vi "snake FGV.vi"(0 "X Step Size":fxp<+/-,32,16>, 1 "X End":fxp<+/-,32,16>, 2 "Det Frequency":fxp<+,32,0>=0.9999999997671694, 3 "Traj Frequency":fxp<+,32,0>=0.9999999997671694, 5 "X Start":fxp<+/-,32,16>, 7 "Action":T2, 9 "Y Start":fxp<+/-,32,16>, 11 "Y Step Size":fxp<+/-,32,16>, 12 "Y End":fxp<+/-,32,16>, 13 "Inner Scan axis":T1) -> (4 "X position":fxp<+/-,32,16>, 6 "Y position":fxp<+/-,32,16>, 10 "Number of positions":u32, 15 "Trajectory Complete":bool)   [LabVIEW 2015]
uses:
  Trajectory FGV states.ctl
  Inner Scan axis.ctl
  <vilib>/rvi/Emulation/niFpgaGetClockAttributes.vi
  <vilib>/rvi/Emulation/niFpgaSctlEmulationGetInTimedLoop.vi
  <vilib>/rvi/Emulation/niFpgaEmulationReportErrorSimple.vi
  <vilib>/rvi/Emulation/niFpgaCriticalErrorInLSC.vi
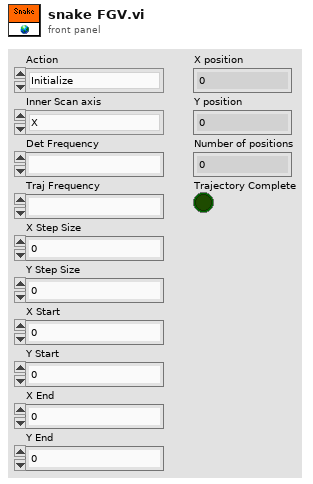
[diagram p1: front panel]
types:
  T1 = typedef "Inner Scan axis.ctl" = enum16{"X", "Y"}
  T2 = typedef "Trajectory FGV states.ctl" = enum16{"Initialize", "Increment"}
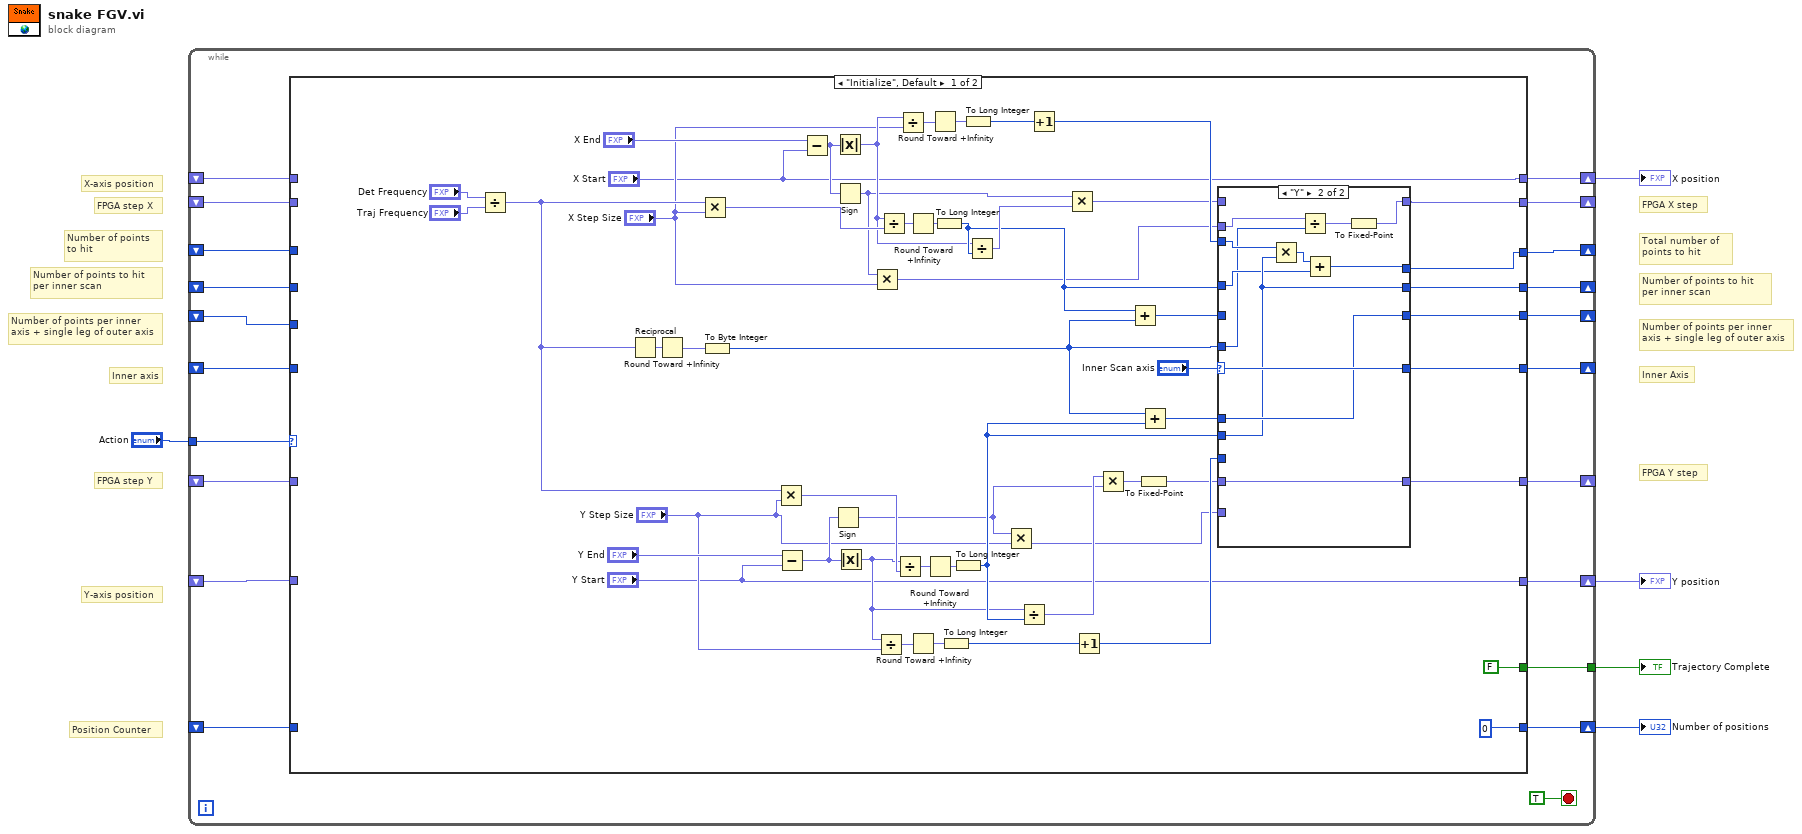
[diagram p0: block diagram]
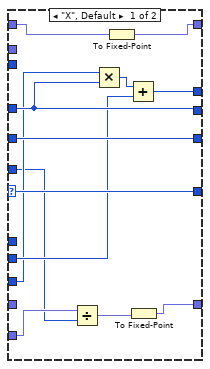
[diagram p2: hidden frame]
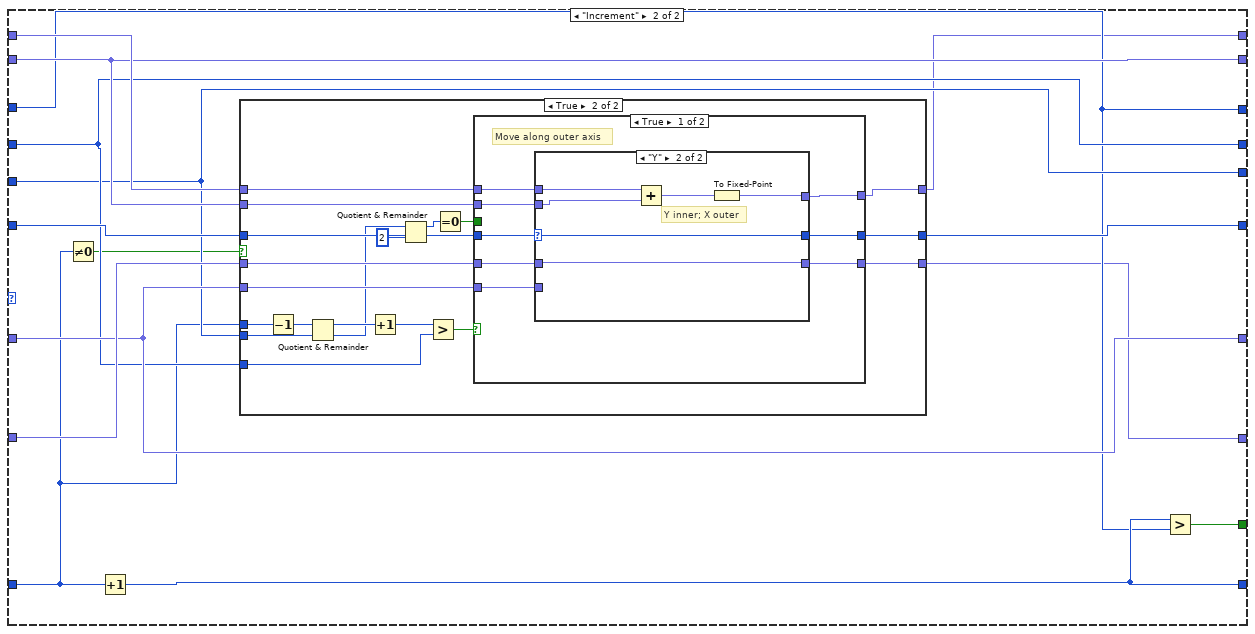
[diagram p3: hidden frame]
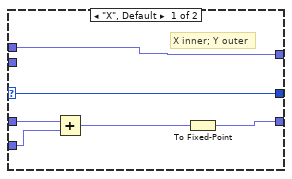
[diagram p5: hidden frame]
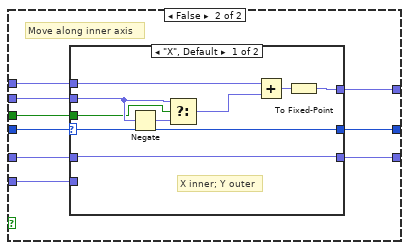
[diagram p6: hidden frame]
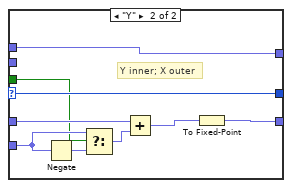
[diagram p7: hidden frame]
diagram:
  # "Number of points per inner \naxis + single leg of outer axis"
  # "Number of points to hit \nper inner scan"
  # "Number of points per inner \naxis + single leg of outer axis"
  # "Inner Axis"
  # "Number of points to hit \nper inner scan"
  # "Inner axis"
  # "FPGA Y step"
  # "FPGA step Y"
  # "Total number of \npoints to hit"
  # "FPGA X step"
  # "Position Counter"
  # "X-axis position"
  # "Y-axis position"
  # "FPGA step X"
  # "Number of points\nto hit"
  n1 = while {
    tunnel: "Action" -> [w25]
    shift-right: [w18] -> _
    shift-left: _ -> [w23]
    shift-right: [w22] -> _
    shift-left: _ -> [w15]
    shift-right: [w6] -> w2
    shift-left: _ -> [w24]
    tunnel: [w21] -> w4
    shift-right: [w20] -> w3
    shift-left: _ -> [w19]
    shift-right: [w17] -> _
    shift-left: _ -> [w16]
    shift-right: [w14] -> _
    shift-left: _ -> [w13]
    shift-right: [w11] -> _
    shift-left: _ -> [w12]
    shift-right: [w10] -> _
    shift-left: _ -> [w9]
    shift-right: [w8] -> w1
    shift-left: _ -> [w7]
    stop <- TRUE stop-if-true
    n2 = case shown="\"Initialize\", Default" w25 {
      tunnel: w7 -> [_ w116]
      tunnel: w24 -> [_ w115]
      tunnel: w23 -> [_ w113]
      tunnel: [w39 w112] -> w17
      tunnel: [w51 w106] -> w22
      tunnel: [FALSE w118] -> w21
      tunnel: [u32 0 w107] -> w20
      tunnel: w19 -> [_ w108]
      tunnel: [w37 w113] -> w18
      tunnel: w16 -> [_ w112]
      tunnel: w15 -> [_ w106]
      tunnel: [w66 w114] -> w14
      tunnel: w13 -> [_ w117]
      tunnel: w12 -> [_ w110]
      tunnel: [w63 w110] -> w11
      tunnel: [w62 w111] -> w10
      tunnel: w9 -> [_ w111]
      tunnel: ["X Start" w105] -> w8
      tunnel: ["Y Start" w104] -> w6
      frame "Initialize", Default {
        n3 = Divide(x="Det Frequency", y="Traj Frequency") -> (x/y=w61:fxp<+,24,8>)
        n4 = Reciprocal(x=w61) -> (1/x=w69:fxp<+,25,17>)
        n5 = Round Toward +Infinity(x=w69) -> (ceil(x): smallest int >= x=w68:fxp<+,17,17>)
        n6 = Multiply(x=w61, y="X Step Size") -> (x*y=w57:fxp<+/-,56,24>)
        n7 = To Byte Integer(number=w68) -> (8bit integer=w34:i8)
        n8 = Multiply(x=w61, y="Y Step Size") -> (x*y=w59:fxp<+/-,56,24>)
        n9 = Subtract(x="Y End", y="Y Start") -> (x-y=w54:fxp<+/-,33,17>)
        n10 = Subtract(x="X End", y="X Start") -> (x-y=w56:fxp<+/-,33,17>)
        n11 = Sign(1:w54) -> (0:w29:fxp<+/-,2,2>)
        n12 = Absolute Value(x=w56) -> (abs(x)=w44:fxp<+,32,16>)
        n13 = Sign(1:w56) -> (0:w27:fxp<+/-,2,2>)
        n14 = Absolute Value(x=w54) -> (abs(x)=w50:fxp<+,32,16>)
        n15 = Multiply(x=w27, y="X Step Size") -> (x*y=w28:fxp<+/-,33,17>)
        n16 = Divide(x=w50, y="Y Step Size") -> (x/y=w49:fxp<+/-,64,33>)
        n17 = Divide(x=w44, y=w57) -> (x/y=w73:fxp<+/-,64,49>)
        n18 = Divide(x=w50, y=w59) -> (x/y=w74:fxp<+/-,64,49>)
        n19 = Divide(x=w44, y="X Step Size") -> (x/y=w46:fxp<+/-,64,33>)
        n20 = Round Toward +Infinity(x=w73) -> (ceil(x): smallest int >= x=w72:fxp<+/-,50,50>)
        n21 = Round Toward +Infinity(x=w49) -> (ceil(x): smallest int >= x=w48:fxp<+/-,34,34>)
        n22 = Round Toward +Infinity(x=w74) -> (ceil(x): smallest int >= x=w60:fxp<+/-,50,50>)
        n23 = Round Toward +Infinity(x=w46) -> (ceil(x): smallest int >= x=w45:fxp<+/-,34,34>)
        n24 = To Long Integer(number=w72) -> (32bit integer=w53:i32)
        n25 = To Long Integer(number=w48) -> (32bit integer=w47:i32)
        n26 = To Long Integer(number=w60) -> (32bit integer=w52:i32)
        n27 = To Long Integer(number=w45) -> (32bit integer=w43:i32)
        n28 = Divide(x=w44, y=w53) -> (x/y=w55:fxp<+/-,64,17>)
        n29 = Multiply(x=w29, y="Y Step Size") -> (x*y=w30:fxp<+/-,33,17>)
        n30 = Divide(x=w50, y=w52) -> (x/y=w58:fxp<+/-,64,17>)
        n31 = Increment(x=w43) -> (x+1=w42:i32)
        n32 = Multiply(x=w27, y=w55) -> (x*y=w38:fxp<+/-,64,18>)
        n33 = Increment(x=w47) -> (x+1=w41:i32)
        n34 = Multiply(x=w58, y=w29) -> (x*y=w40:fxp<+/-,64,18>)
        n35 = Add(x=w53, y=w34) -> (x+y=w65:i32)
        n36 = To Fixed-Point(number=w40) -> (fixed-point=w32:fxp<+/-,24,16>)  [unwired: 1 in]
        n37 = Add(x=w34, y=w52) -> (x+y=w64:i32)
        n38 = case shown="\"Y\"" "Inner Scan axis" {
          selector: "Inner Scan axis" -> [w90 w103]
          tunnel: [w90 w103] -> w66
          tunnel: w65 -> [w91 _]
          tunnel: w64 -> [_ w102]
          tunnel: [w91 w102] -> w63
          tunnel: w52 -> [w86 w100]
          tunnel: w53 -> [w88 w99]
          tunnel: [w88 w100] -> w62
          tunnel: [w87 w97] -> w51
          tunnel: w41 -> [w85 _]
          tunnel: w42 -> [_ w98]
          tunnel: w32 -> [_ w96]
          tunnel: [w81 w96] -> w39
          tunnel: w38 -> [w80 _]
          tunnel: [w79 w92] -> w37
          tunnel: w30 -> [w84 _]
          tunnel: w28 -> [_ w95]
          tunnel: w34 -> [w83 w94]
          frame "X", Default {
            n39 = Divide(x=w84, y=w83) -> (x/y=w82:fxp<+/-,41,17>)
            n40 = Multiply(x=w85, y=w88) -> (x*y=w89:i32)
            n41 = To Fixed-Point(number=w80) -> (fixed-point=w79:fxp<+/-,24,16>)  [unwired: 1 in]
            n42 = Add(x=w89, y=w86) -> (x+y=w87:i32)
            n43 = To Fixed-Point(number=w82) -> (fixed-point=w81:fxp<+/-,24,16>)  [unwired: 1 in]
          }
          frame "Y" {
            n44 = Multiply(x=w98, y=w100) -> (x*y=w101:i32)
            n45 = Divide(x=w95, y=w94) -> (x/y=w93:fxp<+/-,41,17>)
            n46 = Add(x=w101, y=w99) -> (x+y=w97:i32)
            n47 = To Fixed-Point(number=w93) -> (fixed-point=w92:fxp<+/-,24,16>)  [unwired: 1 in]
          }
        }
      }
      frame "Increment" {
        n48 = Not Equal To 0?(x=w108) -> (x != 0?=w109:bool)
        n49 = Increment(x=w108) -> (x+1=w107:u32)
        n50 = case shown="True" w109 {
          tunnel: w117 -> [w121 w140]
          tunnel: w116 -> [w119 w139]
          tunnel: w115 -> [w120 w138]
          tunnel: [w120 w137] -> w104
          tunnel: [w121 w136] -> w114
          tunnel: w108 -> [_ w135]
          tunnel: w113 -> [_ w132]
          tunnel: w112 -> [_ w131]
          tunnel: w111 -> [_ w126]
          tunnel: w110 -> [_ w127]
          tunnel: [w119 w122] -> w105
          frame False {
          }
          frame True {
            n51 = Decrement(x=w135) -> (x-1=w124:u32)
            n52 = Quotient & Remainder(x=w124, y=w127) -> (x-y*floor(x/y)=w134:u32, floor(x/y)=w125:u32)
            n53 = Increment(x=w134) -> (x+1=w123:u32)
            n54 = Quotient & Remainder(x=w125, y=u32 2) -> (x-y*floor(x/y)=w129:u32)  [unwired: 1 out]
            n55 = Greater?(x=w123, y=w126) -> (0:w133:bool)
            n56 = Equal To 0?(x=w129) -> (x = 0?=w128:bool)
            n57 = case shown="True" w133 {
              tunnel: w140 -> [w148 w169]
              tunnel: w139 -> [w147 w168]
              tunnel: [w141 w167] -> w122
              tunnel: w138 -> [w146 w166]
              tunnel: [w145 w165] -> w137
              tunnel: w131 -> [w144 w164]
              tunnel: w132 -> [w143 w163]
              tunnel: [w142 w162] -> w136
              tunnel: w128 -> [_ w161]
              frame True {
                # "Move along outer axis"
                n58 = case shown="\"Y\"" w148 {
                  selector: w148 -> [w153 w157]
                  tunnel: w147 -> [w151 w160]
                  tunnel: w143 -> [_ w159]
                  tunnel: w146 -> [w154 w158]
                  tunnel: [w149 w158] -> w145
                  tunnel: w144 -> [w152 _]
                  tunnel: [w153 w157] -> w142
                  tunnel: [w151 w155] -> w141
                  frame "X", Default {
                    # "X inner; Y outer"
                    n59 = Add(x=w154, y=w152) -> (x+y=w150:fxp<+/-,33,17>)
                    n60 = To Fixed-Point(number=w150) -> (fixed-point=w149:fxp<+/-,24,16>)  [unwired: 1 in]
                  }
                  frame "Y" {
                    # "Y inner; X outer"
                    n61 = Add(x=w160, y=w159) -> (x+y=w156:fxp<+/-,33,17>)
                    n62 = To Fixed-Point(number=w156) -> (fixed-point=w155:fxp<+/-,24,16>)  [unwired: 1 in]
                  }
                }
              }
              frame False {
                # "Move along inner axis"
                n63 = case shown="\"X\", Default" w169 {
                  selector: w169 -> [w176 w186]
                  tunnel: w168 -> [w178 w181]
                  tunnel: w163 -> [w174 _]
                  tunnel: [w170 w181] -> w167
                  tunnel: w166 -> [w177 w187]
                  tunnel: [w177 w179] -> w165
                  tunnel: w164 -> [_ w185]
                  tunnel: [w176 w186] -> w162
                  tunnel: w161 -> [w172 w184]
                  frame "X", Default {
                    # "X inner; Y outer"
                    n64 = Negate(x=w174) -> (-x=w173:fxp<+/-,25,17>)
                    n65 = Select(t=w174, s=w172, f=w173) -> (s? t:f=w175:fxp<+/-,25,17>)
                    n66 = Add(x=w178, y=w175) -> (x+y=w171:fxp<+/-,33,17>)
                    n67 = To Fixed-Point(number=w171) -> (fixed-point=w170:fxp<+/-,24,16>)  [unwired: 1 in]
                  }
                  frame "Y" {
                    # "Y inner; X outer"
                    n68 = Negate(x=w185) -> (-x=w183:fxp<+/-,25,17>)
                    n69 = Select(t=w185, s=w184, f=w183) -> (s? t:f=w182:fxp<+/-,25,17>)
                    n70 = Add(x=w187, y=w182) -> (x+y=w180:fxp<+/-,33,17>)
                    n71 = To Fixed-Point(number=w180) -> (fixed-point=w179:fxp<+/-,24,16>)  [unwired: 1 in]
                  }
                }
              }
            }
          }
        }
        n72 = Greater?(x=w107, y=w106) -> (0:w118:bool)
      }
    }
  }
  "Number of positions" <- w3
  "X position" <- w1
  "Y position" <- w2
  "Trajectory Complete" <- w4
